vi "SequenceAcquire Callback.vi"(4 "Cluster":T9 {"Config In"."Hardware Configuration"."Lasers Configuration"."SettingValues"."785 Power" format="%.1f"; "Config In"."Hardware Configuration"."Lasers Configuration"."SettingValues"."647 Power" format="%.1f"; "Config In"."Hardware Configuration"."Lasers Configuration"."SettingValues"."561 Power" format="%.1f"}, 5 "Event Data":cluster{"sender":refnum<k24>, "e":refnum<k24>}, 6 "Control Ref":refnum<k24>, 7 "Event Common Data":T10) -> ()   [LabVIEW 2020]
uses:
  D:/Daguan/Development/RM21-MMicrosopeSource/HardwareAdapter/Camera/Dependencies/PVCamNET.dll
  HardwareAdapter/Camera/Dependencies/PVCamNET.dll
  DataQueuesAndNotifier.ctl
  Settings/System Running Settings.ctl
  HardwareAdapter/Support/Hardware Configuration.ctl
  HardwareAdapter/Support/Camera Configuration.ctl
  <vilib>/vision/Image Controls.llb/IMAQ Image.ctl
  D:/Daguan/Development/RM21-MMicrosopeSource/HardwareAdapter/Lasers/Dependencies/Oxxius_Boxx.dll
  HardwareAdapter/Lasers/Dependencies/Oxxius_Boxx.dll
  Logging/Logging Configuration.ctl
  controls/DeviceStatusCtl.ctl
  controls/CallBack Refs.ctl
  controls/Image MatadataCtl.ctl
  Global.vi
  Logging/Logging.lvlib
  Settings/Settings.lvlib
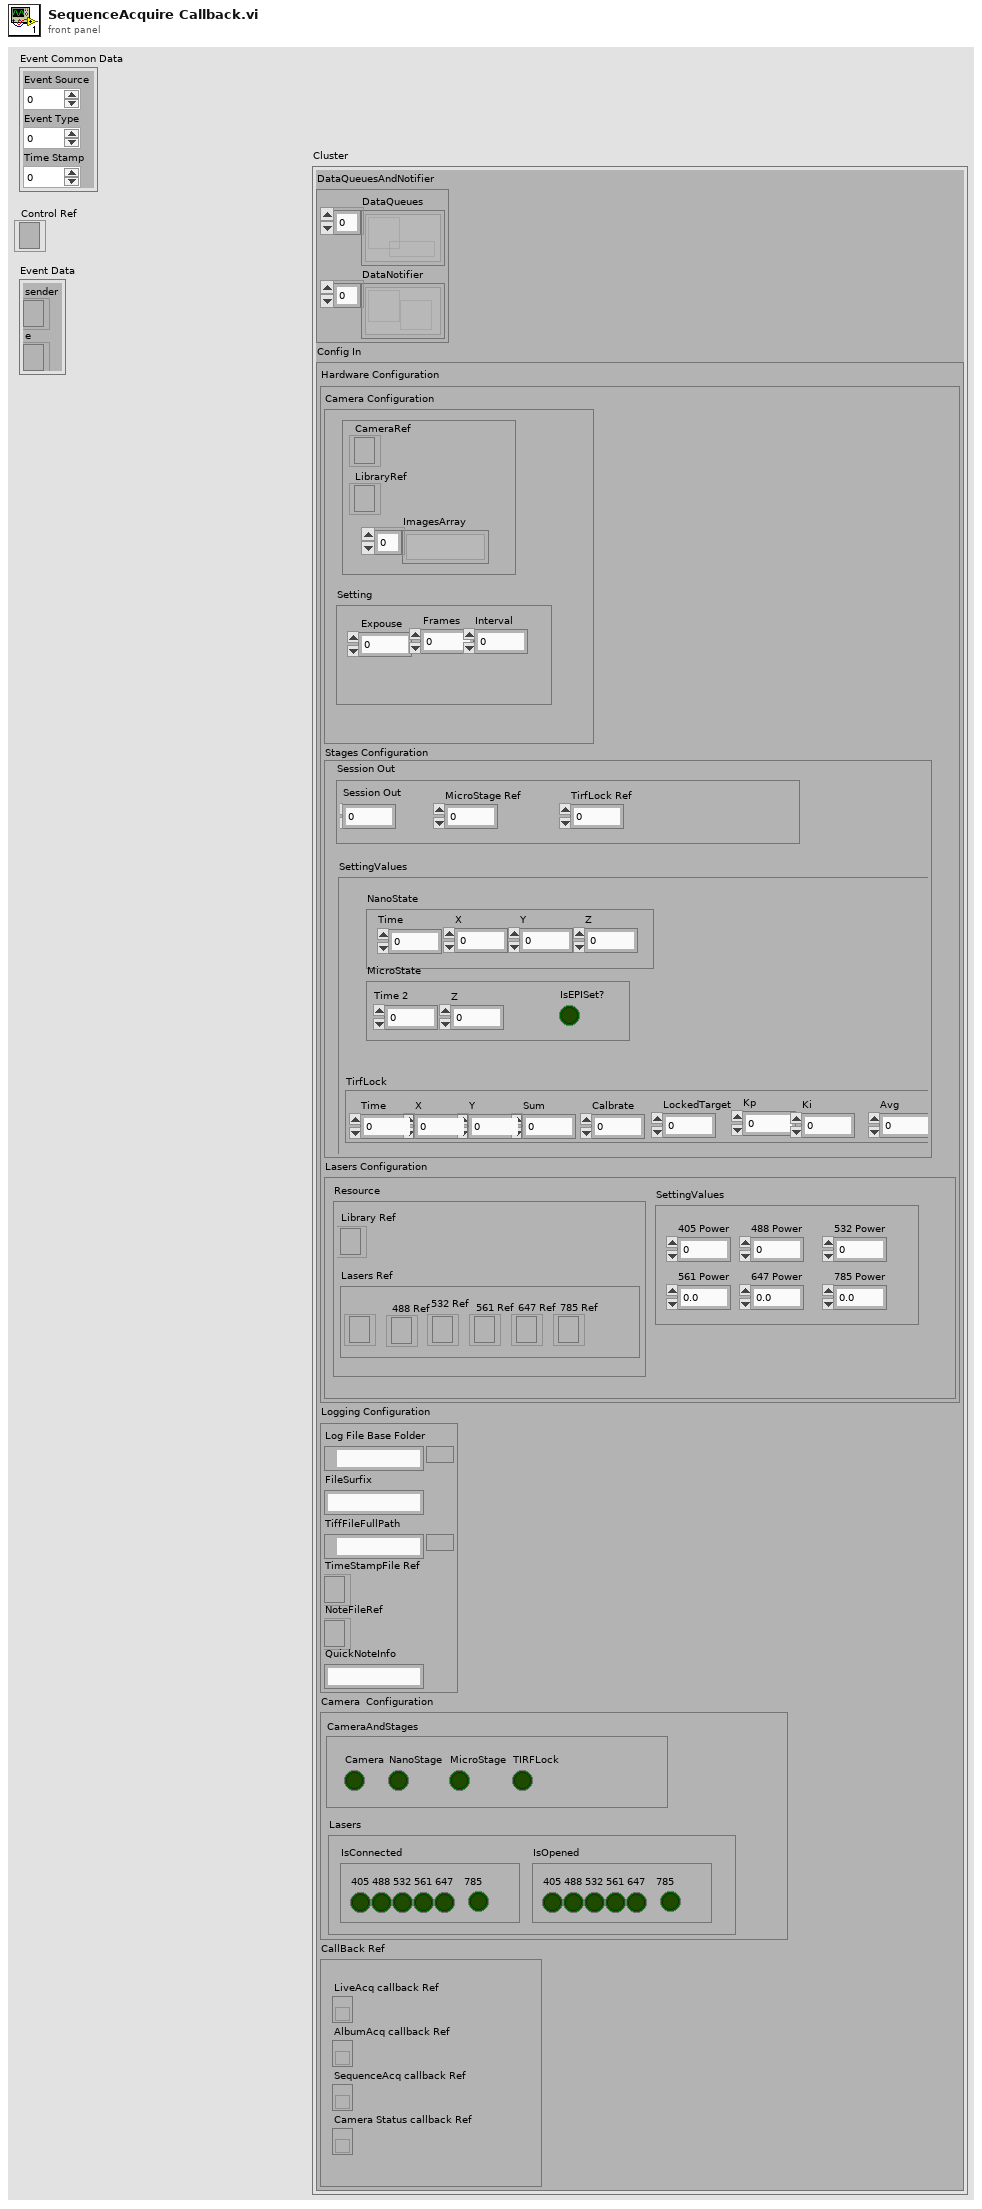
[diagram p1: front panel]
types:
  T1 = typedef "DataQueuesAndNotifier.ctl" = cluster{"DataQueues":refnum<queue>[], "DataNotifier":refnum<notifier>[]}
  T2 = typedef "Settings.lvlib/System Running Settings.ctl" = cluster{"Hardware Configuration":T3, "Logging Configuration":T6, "HardWare Status":cluster{"CameraAndStages":T7, "Lasers":cluster{"IsConnected":cluster{"405":bool, "488":bool, "532":bool, "561":bool, "647":bool, "785":bool}, "IsOpened":cluster{"405":bool, "488":bool, "532":bool, "561":bool, "647":bool, "785":bool}}}, "CallBack Ref":T8}
  T3 = typedef "Hardware Configuration.ctl" = cluster{"Camera Configuration":T4, "Stages Configuration":cluster{"Resource":cluster{"NanoStage Ref":i32, "MicroStage Ref":i32, "TirfLock Ref":i32}, "SettingValues":cluster{"NanoState":cluster{"Time":dbl, "X":dbl, "Y":dbl, "Z":dbl}, "MicroState":cluster{"Time 2":dbl, "Z":dbl, "IsEPISet?":bool}, "TirfLock":cluster{"Time":dbl, "X":dbl, "Y":dbl, "Sum":dbl, "Calbrate":dbl, "LockedTarget":dbl, "Kp":dbl, "Ki":dbl, "Avg":dbl}}}, "Lasers Configuration":cluster{"SettingValues":cluster{"405 Power":sgl, "488 Power":sgl, "532 Power":sgl, "561 Power":sgl, "647 Power":sgl, "785 Power":sgl}, "Resource":cluster{"Library Ref":refnum<k24>, "Lasers Ref":cluster{"405 Ref":refnum<k24>, "488 Ref":refnum<k24>, "532 Ref":refnum<k24>, "561 Ref":refnum<k24>, "647 Ref":refnum<k24>, "785 Ref":refnum<k24>}}}}
  T4 = typedef "Camera Configuration.ctl" = cluster{"Setting":cluster{"Expouse":dbl, "Frames":dbl, "Interval":dbl}, "Resource":cluster{"CameraRef":refnum<k24>, "LibraryRef":refnum<k24>, "ImagesArray":T5[]}}
  T5 = typedef "IMAQ Image.ctl" = refnum<image>
  T6 = typedef "Logging.lvlib/Logging Configuration.ctl" = cluster{"Log File Base Folder":path, "FileSurfix":string, "TiffFileFullPath":path, "TimeStampFile Ref":refnum<file>, "NoteFileRef":refnum<file>, "QuickNoteInfo":string}
  T7 = typedef "DeviceStatusCtl.ctl" = cluster{"Camera":bool, "NanoStage":bool, "MicroStage":bool, "TIRFLock":bool}
  T8 = typedef "CallBack Refs.ctl" = cluster{"LiveAcq callback Ref":refnum<k27>, "AlbumAcq callback Ref":refnum<k27>, "SequenceAcq callback Ref":refnum<k27>, "Camera Status callback Ref":refnum<k27>}
  T9 = cluster{"DataQueuesAndNotifier":T1, "Config In":T2}
  T10 = cluster{"Event Source":i32, "Event Type":u32, "Time Stamp":u32}
  T11 = typedef "Image MatadataCtl.ctl" = cluster{"EofTimeStamp(Acq)":dbl, "Image":T5, "Histogram":u32[], "MeanValue":dbl, "Min":u32, "Max":u32, "EofTimeStamp(Album)":dbl, "Fps":dbl, "BufferIndex":u32, "DroppedFrames":u32, "SaveImage?":bool}
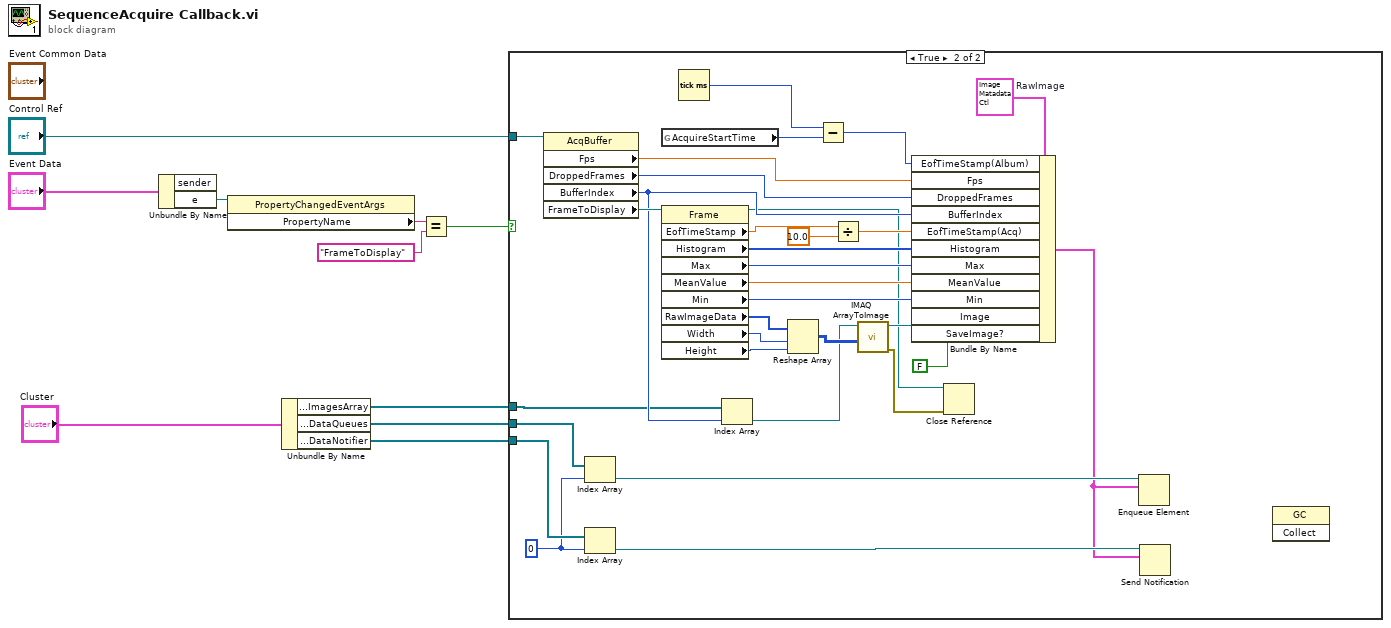
[diagram p0: block diagram]
diagram:
  n1 = Unbundle By Name("Event Data") -> ("e"=w9:refnum<k24>)  [unwired: 1 out]
  n2 = property class="PropertyChangedEventArgs"(reference=w9) -> ("PropertyName"=w8:string)  [unwired: 1 in, 2 out]
  n3 = Unbundle By Name("Cluster") -> ("Config In.Hardware Configuration.Camera Configuration.Resource.ImagesArray"=w3:T5[], "DataQueuesAndNotifier.DataQueues"=w2:refnum<queue>[], "DataQueuesAndNotifier.DataNotifier"=w1:refnum<notifier>[])
  n4 = Equal?(x=w8, y="FrameToDisplay") -> (x = y?=w6:bool)
  n5 = case shown="True" w6 {
    tunnel: "Control Ref" -> [_ w42]
    tunnel: w3 -> [_ w24]
    tunnel: w2 -> [_ w22]
    tunnel: w1 -> [_ w21]
    frame False {
    }
    frame True {
      w20 = 0 ("index")
      w31 = T11 {"EofTimeStamp(Acq)"=0.0, "Image"=refnum, "Histogram"=[], "MeanValue"=0.0, "Min"=0, "Max"=0, "EofTimeStamp(Album)"=0.0, "Fps"=0.0, "BufferIndex"=0, "DroppedFrames"=0, "SaveImage?"=FALSE}  # RawImage
      n6 = property class="AcqBuffer"(reference=w42) -> ("Fps"=w27:sgl, "DroppedFrames"=w26:i32, "BufferIndex"=w25:i32, "FrameToDisplay"=w41:refnum<k24>)  [unwired: 1 in, 2 out]
      n7 = Index Array(array=w22, index=w20) -> (element=w19:refnum<queue>)
      n8 = Index Array(array=w21, index=w20) -> (element=w18:refnum<notifier>)
      n9 = global read "Global.vi" "AcquireStartTime"() -> (w15:u32)
      n10 = property class="Frame"(reference=w41) -> (reference out=w13:refnum<k24>, "EofTimeStamp"=w28:dbl, "Histogram"=w32:u32[], "Max"=w33:u32, "MeanValue"=w34:dbl, "Min"=w37:u32, "RawImageData"=w38:i16[], "Width"=w40:u32, "Height"=w39:u32)  [unwired: 1 in, 1 out]
      n11 = Tick Count (ms)() -> (millisecond timer value=w16:u32)
      n12 = Index Array(array=w24, index=w25) -> (element=w23:T5)
      n13 = Reshape Array "Reshape Array"(w38, w40, w39) -> (w36:i16[][])
      n14 = Subtract(x=w16, y=w15) -> (x-y=w14:u32)
      n15 = Divide(x=w28, y=10.0) -> (x/y=w29:dbl)
      n16 = call "IMAQ ArrayToImage"("Image Pixels (I16)"=w36, "Image"=w23) -> ("error out"=w12:errorcluster, "Image Out"=w35:T5)  [unwired: 8 in]
      n17 = Bundle By Name(cluster=w31, "EofTimeStamp(Album)"=w14, "Fps"=w27, "DroppedFrames"=w26, "BufferIndex"=w25, "EofTimeStamp(Acq)"=w29, "Histogram"=w32, "Max"=w33, "MeanValue"=w34, "Min"=w37, "Image"=w35, "SaveImage?"=FALSE) -> (w17:T11)
      n18 = Close Reference(reference=w13, error in (no error)=w12) -> ()  [unwired: 1 out]
      n19 = Enqueue Element(queue=w19, element=w17) -> ()  [unwired: 2 in, 3 out]
      n20 = Send Notification(notification=w17, notifier=w18) -> ()  [unwired: 1 in, 2 out]
      n21 = invoke class="GC" method="Collect"() -> ()  [unwired: 3 in, 3 out]
    }
  }
